vi "datosTraspaso_to_Arduino.vi"(8 "error in (no error)":errorcluster, 9 "TRASPASO ASICS INPUT":T1={"COORD X ORIGEN"=0, "COORD  Y ORIGEN"=0, "NºASICS A MOVER"=1, "BANDEJA ORIGEN"=enum."BANDEJA ENTRADA", "BANDEJA DESTINO"=enum."BANDEJA ENTRADA", "COORD X DESTINO "=0, "COORD  Y DESTINO "=0, "CONTEO TRASLADOS"=0}, 11 "VISA resource name":refnum<visa-resource-name>) -> (0 "error IO":errorcluster, 2 "trama datos devuelta":string, 3 "trama datos enviada":string)   [LabVIEW 2019]
uses:
  TYPE'S DEF/INPUT_TRASPASO_ASICS.ctl
  <vilib>/Utility/error.llb/Error Cluster From Error Code.vi
  <vilib>/ErrorRing/Error Ring.xnode
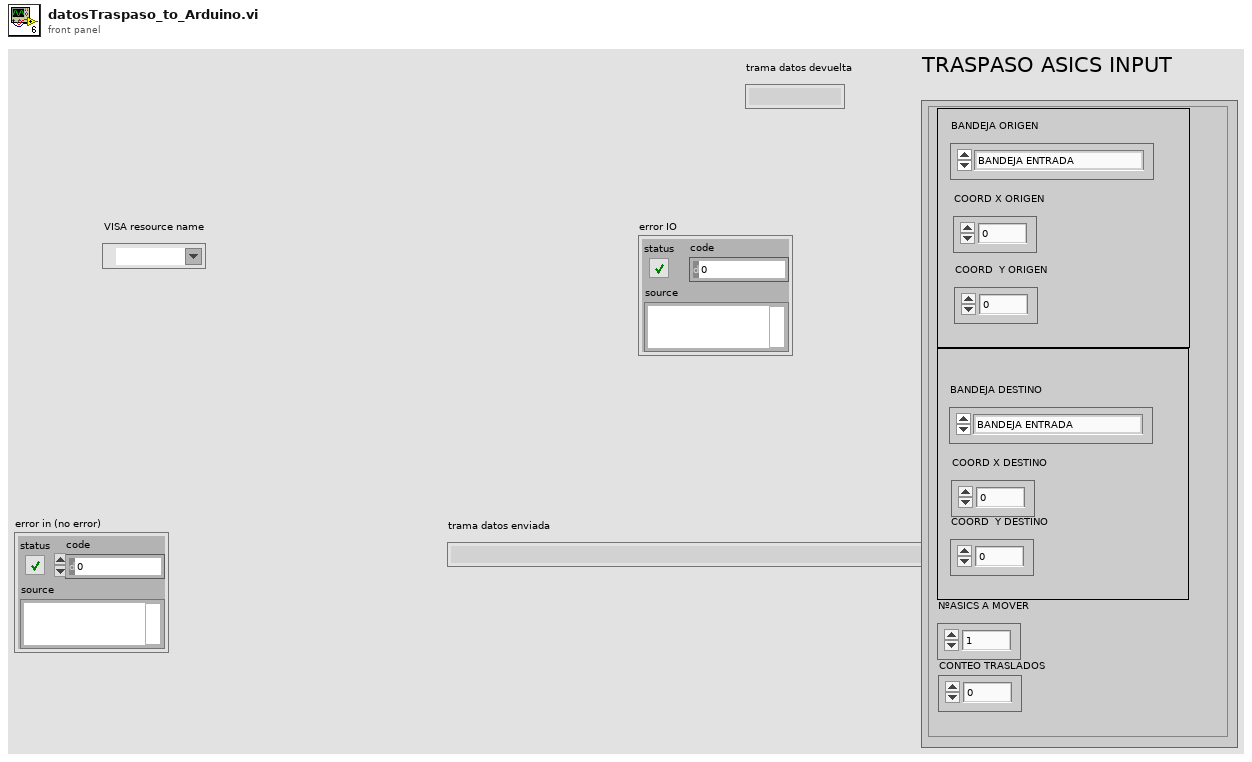
[diagram p1: front panel]
types:
  T1 = typedef "INPUT_TRASPASO_ASICS.ctl" = cluster{"COORD X ORIGEN":u32, "COORD  Y ORIGEN":u32, "NºASICS A MOVER":u32, "BANDEJA ORIGEN":enum16{"BANDEJA ENTRADA", "BANDEJA OK", "BANDEJA NOK"}, "BANDEJA DESTINO":enum16{"BANDEJA ENTRADA", "BANDEJA OK", "BANDEJA NOK"}, "COORD X DESTINO ":u32, "COORD  Y DESTINO ":u32, "CONTEO TRASLADOS":u32}
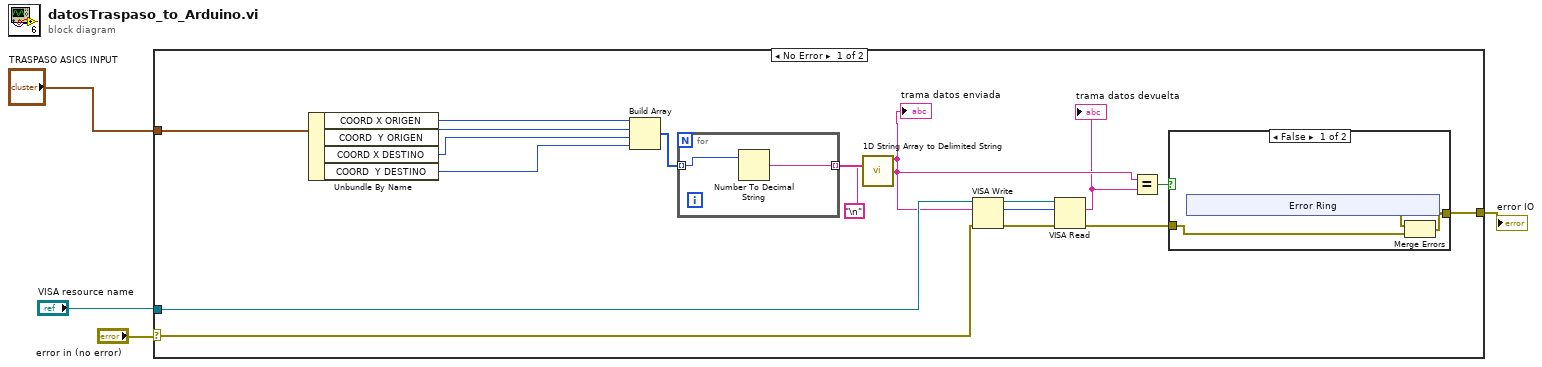
[diagram p0: block diagram]
diagram:
  n1 = case shown="No Error" "error in (no error)" {
    selector: "error in (no error)" -> [w18 w34]
    tunnel: "VISA resource name" -> [w19 _]
    tunnel: [w11 w34] -> w2
    tunnel: "TRASPASO ASICS INPUT" -> [w7 _]
    frame No Error {
      n2 = Unbundle By Name(w7) -> ("COORD X ORIGEN"=w9:u32, "COORD  Y ORIGEN"=w8:u32, "COORD X DESTINO"=w6:u32, "COORD  Y DESTINO"=w5:u32)
      n3 = Build Array(w9, w8, w6, w5) -> (w22:u32[])
      n4 = for {
        tunnel: w22 -> [w32] mode=indexing
        tunnel: [w33] -> w21 mode=indexing
        n5 = Number To Decimal String(number=w32) -> (decimal integer string=w33:string)  [unwired: 1 in]
      }
      n6 = call <vilib>:"1D String Array to Delimited String.vi"("delimiter"="\n", "string array"=w21) -> ("delimited string"=w14:string)  [unwired: 9 in]
      "trama datos enviada" <- w14
      n7 = VISA Write(VISA resource name=w19, write buffer=w14, error in (no error)=w18) -> (VISA resource name out=w16:refnum<visa-resource-name>, return count=w15:u32, error out=w17:errorcluster)
      n8 = VISA Read(VISA resource name=w16, byte count=w15, error in (no error)=w17) -> (read buffer=w13:string, error out=w10:errorcluster)  [unwired: 2 out]
      "trama datos devuelta" <- w13
      n9 = Equal?(x=w14, y=w13) -> (x = y?=w12:bool)
      n10 = case shown="False" w12 {
        tunnel: [w25 w31] -> w11
        tunnel: w10 -> [w23 w31]
        frame False {
          n11 = xnode "Error Ring"() -> ("error out"=w24:errorcluster)
          n12 = Merge Errors(w24, w23) -> (w25:errorcluster)
        }
        frame True {
        }
      }
    }
    frame Error {
    }
  }
  "error IO" <- w2
